vi "Sampling Frequency.vi"() -> (0 "Sampling Frequency":dbl)   [LabVIEW 2013]
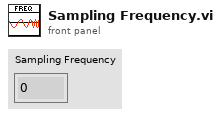
[diagram p1: front panel]
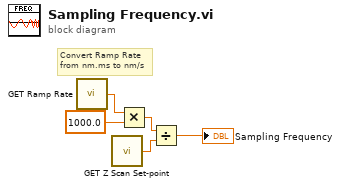
[diagram p0: block diagram]
diagram:
  # "Convert Ramp Rate from nm.ms to nm/s"
  n1 = call "GET Ramp Rate.vi"() -> ("Ramp Rate"=w5:dbl)
  n2 = call "GET Z Scan Set-point.vi"() -> ("Z Scan Set-point"=w2:dbl)
  n3 = Multiply(x=w5, y=1000.0) -> (x*y=w3:dbl)
  n4 = Divide(x=w3, y=w2) -> (x/y=→"Sampling Frequency":dbl)
